vi "time_array_2.vi"() -> ()   [LabVIEW 2017]
panel:
  out "最近10筆大於0.9":dbl[][](array[numeric])
  out "Output":dbl[][](array[numeric])
  out "real time":dbl[](array[numeric])
  out "Waveform Chart":dbl(graph)
  out "day":dbl(knob) scale=0.0..10.0
  out "hr":dbl(knob) scale=0.0..10.0
  out "min":dbl(knob) scale=0.0..60.0
  out "ii":i32
  in  "stop":bool
  out "s":dbl(knob) scale=0.0..60.0
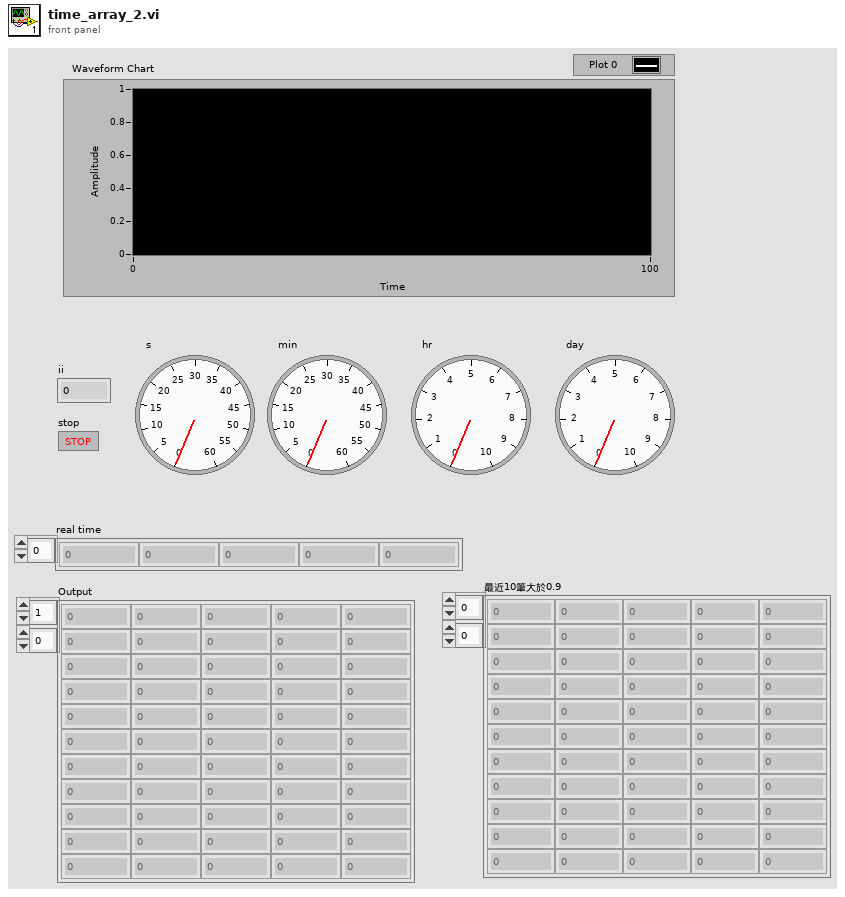
[diagram p1: front panel]
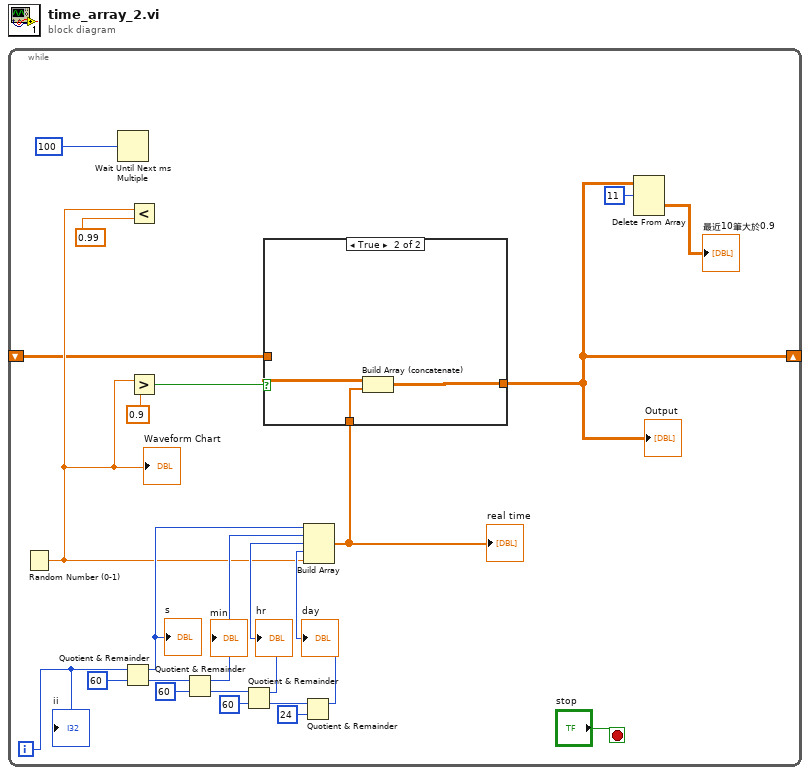
[diagram p0: block diagram]
diagram:
  n1 = while {
    shift-right: [w4] -> _
    shift-left: _ -> [w5]
    i -> [w21]
    stop <- "stop" stop-if-true
    n2 = Random Number (0-1)() -> (number: 0 to 1=w8:dbl)
    "Waveform Chart" <- w8
    n3 = Wait Until Next ms Multiple(millisecond multiple=100) -> ()  [unwired: 1 out]
    n4 = Quotient & Remainder(x=w21, y=60) -> (x-y*floor(x/y)=w12:i32, floor(x/y)=w19:i32)
    "s" <- w12
    n5 = Less?(x=w8, y=0.99) -> ()  [unwired: 1 out]
    n6 = Greater?(x=w8, y=0.9) -> (0:w1:bool)
    n7 = Quotient & Remainder(x=w19, y=60) -> (x-y*floor(x/y)=w11:i32, floor(x/y)=w17:i32)
    "min" <- w11
    n8 = Quotient & Remainder(x=w17, y=60) -> (x-y*floor(x/y)=w10:i32, floor(x/y)=w15:i32)
    "hr" <- w10
    n9 = Quotient & Remainder(x=w15, y=24) -> (x-y*floor(x/y)=w9:i32)  [unwired: 1 out]
    "day" <- w9
    n10 = Build Array(w12, w11, w10, w9, w8) -> (w6:dbl[])
    "real time" <- w6
    n11 = case shown="True" w1 {
      tunnel: w6 -> [_ w26]
      tunnel: w5 -> [w24 w27]
      tunnel: [w24 w25] -> w4
      frame False {
      }
      frame True {
        n12 = Build Array (concatenate)(w27, w26) -> (w25:dbl[][])
      }
    }
    "Output" <- w4
    n13 = Delete From Array(array=w4, length=11) -> (deleted portion=→"最近10筆大於0.9":dbl[][])  [unwired: 2 in, 1 out]
    "ii" <- w21
  }
